vi "Fast_slow loop_property node.vi"() -> ()   [LabVIEW 2010]
panel:
  in  "Stop Loop 2":bool
  out "Loop 2 Iteration Rate (Hz)":dbl
  out "Loop 1 Iteration Rate (Hz)":dbl
  in  "Stop Loop 1":bool
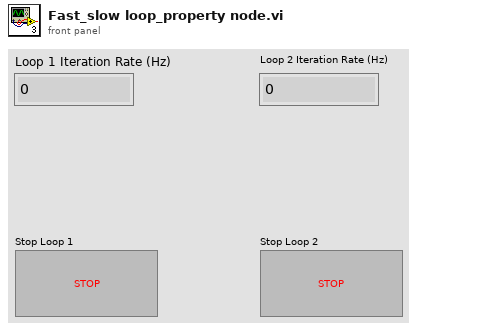
[diagram p1: front panel]
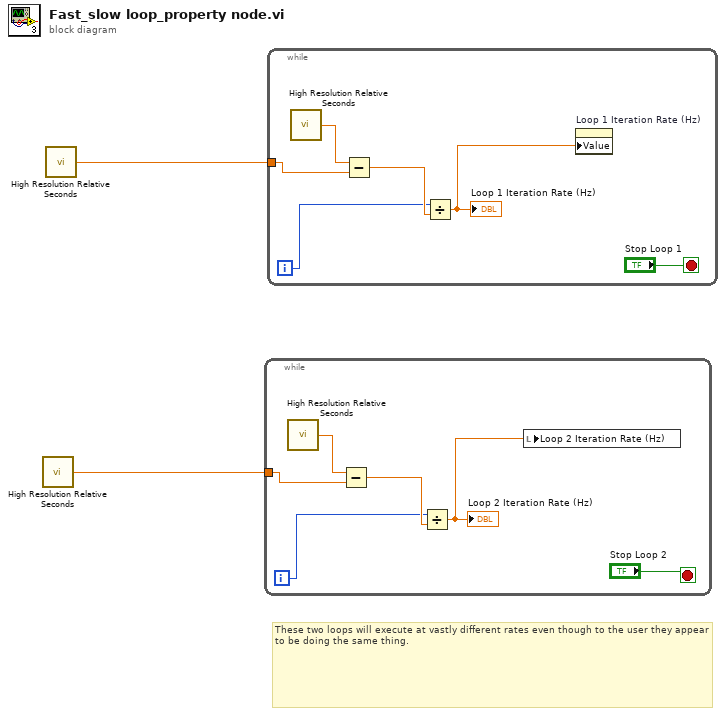
[diagram p0: block diagram]
diagram:
  # "These two loops will execute at vastly different rates even though to the user they appear to be doing the same thing."
  n1 = call <vilib>:"High Resolution Relative Seconds.vi"() -> ("relative seconds"=w2:dbl)
  n2 = call <vilib>:"High Resolution Relative Seconds.vi"() -> ("relative seconds"=w1:dbl)
  n3 = while {
    tunnel: w2 -> [w6]
    i -> [w5]
    stop <- "Stop Loop 2" stop-if-true
    n4 = call <vilib>:"High Resolution Relative Seconds.vi"() -> ("relative seconds"=w7:dbl)
    n5 = Subtract(x=w7, y=w6) -> (x-y=w8:dbl)
    n6 = Divide(x=w5, y=w8) -> (x/y=w3:dbl)
    "Loop 2 Iteration Rate (Hz)" <- w3
    n7 = local write "Loop 2 Iteration Rate (Hz)"(w3) -> ()
  }
  n8 = while {
    tunnel: w1 -> [w11]
    i -> [w10]
    stop <- "Stop Loop 1" stop-if-true
    n9 = call <vilib>:"High Resolution Relative Seconds.vi"() -> ("relative seconds"=w12:dbl)
    n10 = Subtract(x=w12, y=w11) -> (x-y=w13:dbl)
    n11 = Divide(x=w10, y=w13) -> (x/y=w9:dbl)
    "Loop 1 Iteration Rate (Hz)" <- w9
    n12 = property on="Loop 1 Iteration Rate (Hz)" class="DigNum (strict)"("Value"=w9) -> ()  [unwired: 2 in, 2 out]
  }
